vi "Rinocloud_ancestors_to_path.vi"(2 "ancestor array":T1(array[cluster]), 3 "Path":path) -> (1 "full path":path)   [LabVIEW 2013]
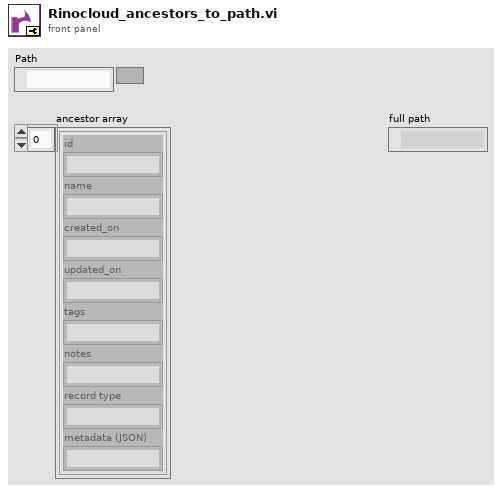
[diagram p1: front panel]
types:
  T1 = cluster{"id":string, "name":string, "created_on":string, "updated_on":string, "tags":string, "notes":string, "record type":string, "metadata (JSON)":string}[]
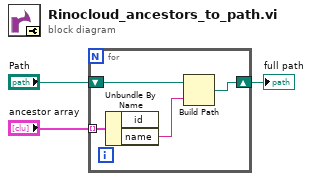
[diagram p0: block diagram]
diagram:
  n1 = for {
    tunnel: "ancestor array" -> [w7] mode=indexing
    shift-right: [w4] -> w1
    shift-left: "Path" -> [w6]
    n2 = Unbundle By Name(w7) -> ("name"=w5:string)  [unwired: 1 out]
    n3 = Build Path(base path=w6, name or relative path=w5) -> (appended path=w4:path)
  }
  "full path" <- w1
